vi "String Contains Polymorphic.vi"   [LabVIEW 2016]
doc: "This Polymorphic VI search a string for a supplied regular expression. This Polymorphic VI can also search an array of string for a specific text."
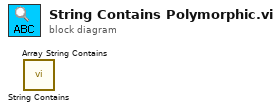
[diagram p0: block diagram]
diagram:
  n1 = call "String Contains.vi"() -> ()  [unwired: 4 in, 2 out]
  n2 = call "Array String Contains.vi"() -> ()  [unwired: 4 in, 2 out]
